vi "grayToColor_test.vi"() -> ()   [LabVIEW 2014]
panel:
  out "2D U32 array":u32[][](array[numeric])
  out "Image 2":T1(plugin-control)
  out "Image":T1(plugin-control)
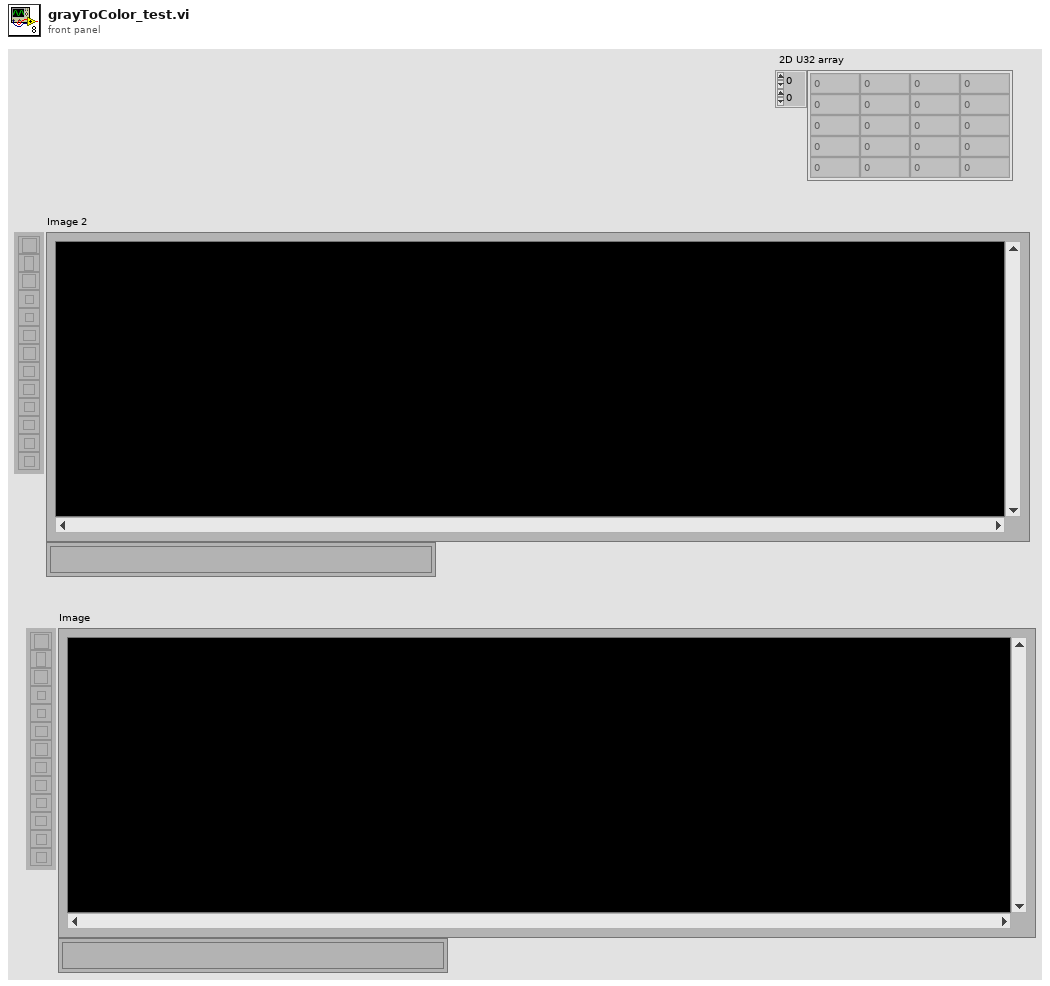
[diagram p1: front panel]
types:
  T1 = typedef "IMAQ Image.ctl" = refnum<image>
  T2 = typedef "Image Type" = u32
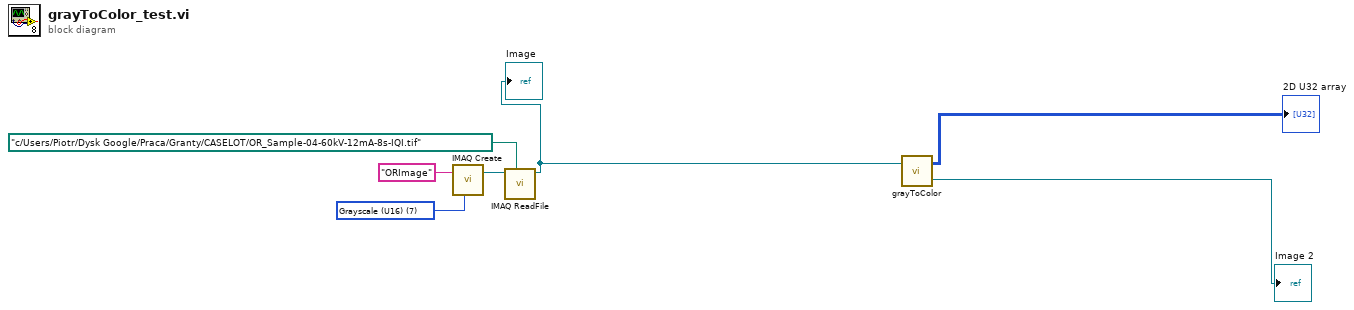
[diagram p0: block diagram]
diagram:
  w6 = T2 7 items=["Grayscale (U8)", "Grayscale (I16)", "Grayscale (SGL)", "Complex (CSG)", "RGB (U32)", "HSL (U32)", "RGB (U64)", "Grayscale (U16)"] ("Image Type")
  n1 = call "IMAQ Create"("Image Name"="ORImage", "Image Type"=w6) -> ("New Image"=w5:T1)  [unwired: 3 in, 1 out]
  n2 = call "IMAQ ReadFile"("File Path"=path "c:/Users/Piotr/Dysk Google/Praca/Granty/CASELOT/OR_Sample-04-60kV-12mA-8s-IQI.tif", "Image"=w5) -> ("Image Out"=w3:T1)  [unwired: 5 in, 4 out]
  "Image" <- w3
  n3 = call "grayToColor.vi"("U16 Image"=w3) -> ("RGB Image"=→"Image 2":T1, "RGB array"=→"2D U32 array":u32[][])  [unwired: 1 in]
